vi "Query To Url Encoded Content.vi"(8 "error in (no error)":errorcluster, 11 "Query":T1) -> (0 "error out":errorcluster, 3 "Url Encoded Content":string)   [LabVIEW 2018, in "InfluxDB Client.lvlib" / "Client.lvclass"]
uses:
  Client.lvclass
  <userlib>/_OpenG.lib/dictionary/dictionary.llb/Dictionary Object RefNum__ogtk.ctl
  <userlib>/_OpenG.lib/dictionary/dictionary.llb/Dictionary Object RefNum - Enum__ogtk.ctl
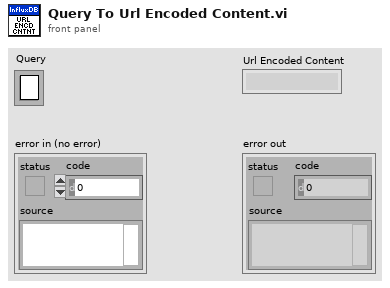
[diagram p1: front panel]
types:
  T1 = typedef "Dictionary Object RefNum__ogtk.ctl" = refnum<k1>
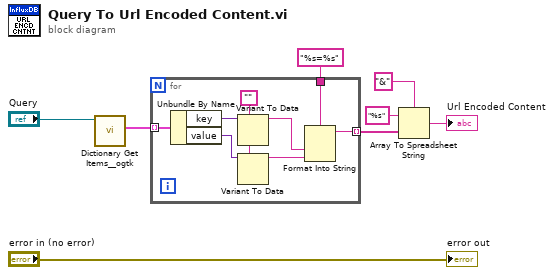
[diagram p0: block diagram]
diagram:
  n1 = call <userlib>:"Dictionary Get Items__ogtk.vi"("dictionary"="Query") -> ("items"=w2:cluster{"key":variant, "value":variant}[])  [unwired: 8 in, 2 out]
  n2 = for {
    tunnel: w2 -> [w14] mode=indexing
    tunnel: "%s=%s" ("format string") -> [w12]
    tunnel: [w9] -> w6 mode=indexing
    w13 = ""
    n3 = Unbundle By Name(w14) -> ("key"=w16:variant, "value"=w15:variant)
    n4 = Variant To Data(type=w13, Variant=w16) -> (data=w11:string)  [unwired: 1 in, 1 out]
    n5 = Variant To Data(type=w13, Variant=w15) -> (data=w10:string)  [unwired: 1 in, 1 out]
    n6 = Format Into String(format string=w12, w11, w10) -> (resulting string=w9:string)  [unwired: 2 in, 1 out]
  }
  n7 = Array To Spreadsheet String(delimiter (Tab)="&", array=w6, 3:"%s" ("format string")) -> (spreadsheet string=→"Url Encoded Content":string)
  "error out" <- "error in (no error)"
